vi "Initiate_Interface.vi"() -> (0 "DLL-Path":path, 1 "instanceHandle":u32, 2 "Fehler (Ausgang)":errorcluster)   [LabVIEW 2016]
uses:
  Utility/Global Constants.vi
  Program Files/MicroEpsilon/MEDAQLib-3.2.3.19901/Samples/LabView/MEDAQLib/MEDAQLib.lvlib
panel:
  out "Error Scale":i32
  out "ERR_CODE 2":i32
  out "ERR_CODE":i32
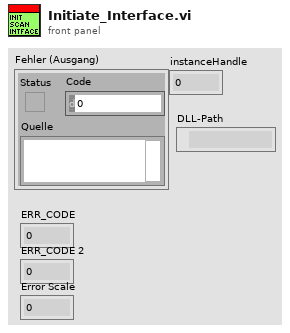
[diagram p1: front panel]
types:
  T1 = enum32{"NONE", "SENSOR_ILD1401", "SENSOR_ILD1700", "SENSOR_ILD1800", "SENSOR_ILD2000", "SENSOR_ILD2200", "SENSOR_IFD2400", "SENSOR_IFD2430", "SENSOR_ODC2500", "SENSOR_ODC2600", "ENCODER_IF2004", "SENSOR_ASP5500", "SENSOR_IFD2401", "SENSOR_IFD2431", "CONTROLLER_ILD1401", "CONTROLLER_DT6500", "SENSOR_DT6100", "CONTROLLER_ESC4912", "CONTROLLER_KSS6380", "SENSOR_ILR110x_115x", "SENSOR_ILR118x", "SENSOR_ILR1191", "PCI_CARD_IF2008", "SENSOR_ILD1402", "SENSOR_ILD1302", "SENSOR_ODC1202", "SENSOR_IFD2471", "CONTROLLER_DT3909", "SENSOR_DT3100", "SENSOR_ILD2300", "SENSOR_IFD2451"}
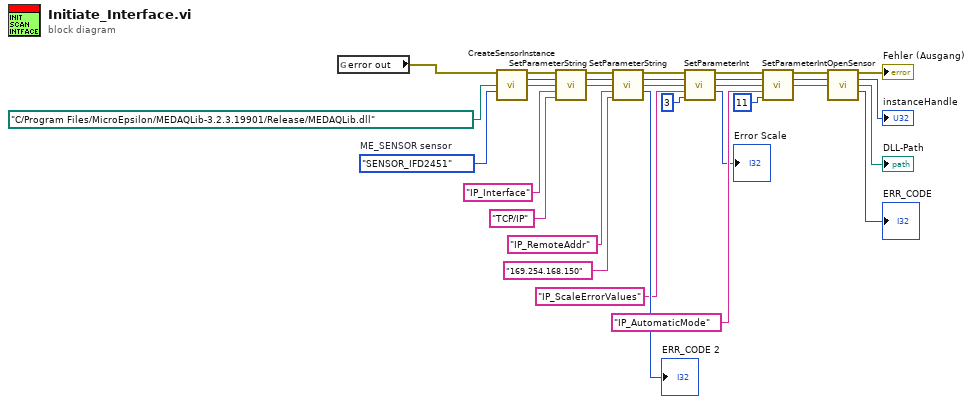
[diagram p0: block diagram]
diagram:
  w12 = T1."SENSOR_IFD2451"  # ME_SENSOR sensor
  n1 = global read "Global Constants.vi" "error out"() -> (w1:errorcluster)
  n2 = call "CreateSensorInstance.vi"("Fehler (Eingang, kein Fehler)"=w1, "DLL-Path"=path "C:/Program Files/MicroEpsilon/MEDAQLib-3.2.3.19901/Release/MEDAQLib.dll", "sensor"=w12) -> ("Fehler (Ausgang)"=w30:errorcluster, "instanceHandle"=w29:u32, "DLL-Path"=w31:path)  [unwired: 10 in]
  n3 = call "SetParameterString.vi"("Fehler (Eingang, kein Fehler)"=w30, "instanceHandle"=w29, "DLL-Path"=w31, "paramName"="IP_Interface", "paramValue"="TCP/IP") -> ("Fehler (Ausgang)"=w21:errorcluster, "instanceHandle"=w20:u32, "DLL-Path"=w19:path)  [unwired: 7 in, 1 out]
  n4 = call "SetParameterString.vi"("Fehler (Eingang, kein Fehler)"=w21, "instanceHandle"=w20, "DLL-Path"=w19, "paramName"="IP_RemoteAddr", "paramValue"="169.254.168.150") -> ("Fehler (Ausgang)"=w5:errorcluster, "instanceHandle"=w6:u32, "DLL-Path"=w7:path, "ERR_CODE"=→"ERR_CODE 2":i32)  [unwired: 7 in]
  n5 = call "SetParameterInt.vi"("Fehler (Eingang, kein Fehler)"=w5, "instanceHandle"=w6, "DLL-Path"=w7, "paramName"="IP_ScaleErrorValues", "paramValue"=3) -> ("Fehler (Ausgang)"=w4:errorcluster, "instanceHandle"=w3:u32, "DLL-Path"=w2:path, "ERR_CODE"=→"Error Scale":i32)  [unwired: 7 in]
  n6 = call "SetParameterInt.vi"("Fehler (Eingang, kein Fehler)"=w4, "instanceHandle"=w3, "DLL-Path"=w2, "paramName"="IP_AutomaticMode", "paramValue"=11) -> ("Fehler (Ausgang)"=w18:errorcluster, "instanceHandle"=w17:u32, "DLL-Path"=w16:path)  [unwired: 7 in, 1 out]
  n7 = call "OpenSensor.vi"("Fehler (Eingang, kein Fehler)"=w18, "instanceHandle"=w17, "DLL-Path"=w16) -> ("Fehler (Ausgang)"=→"Fehler (Ausgang)":errorcluster, "instanceHandle"=→"instanceHandle":u32, "DLL-Path"=→"DLL-Path":path, "ERR_CODE"=→"ERR_CODE":i32)  [unwired: 9 in]
